vi "SE FP hindbrain SENSE.vi"(0 "IR Sensors":T1(array[cluster]), 1 "Analog Input Values":dbl[](array[numeric]), 2 "error in":errorcluster, 4 "GPS":cluster{"X pos":i32, "Y pos":i32, "Heading":dbl}) -> (3 "Boat Status":T2, 5 "error out":errorcluster, 6 "IR Sensors 2":T1(array[cluster]))   [LabVIEW 2014]
doc: "This vi calculate the distance from the boat edge to the detected object. If no object is detected the value is 0. It also determines of the boat is out of power...if so it will stop the boat."
panel:
  out "RIO BAT":dbl
  out "MOT BAT":dbl
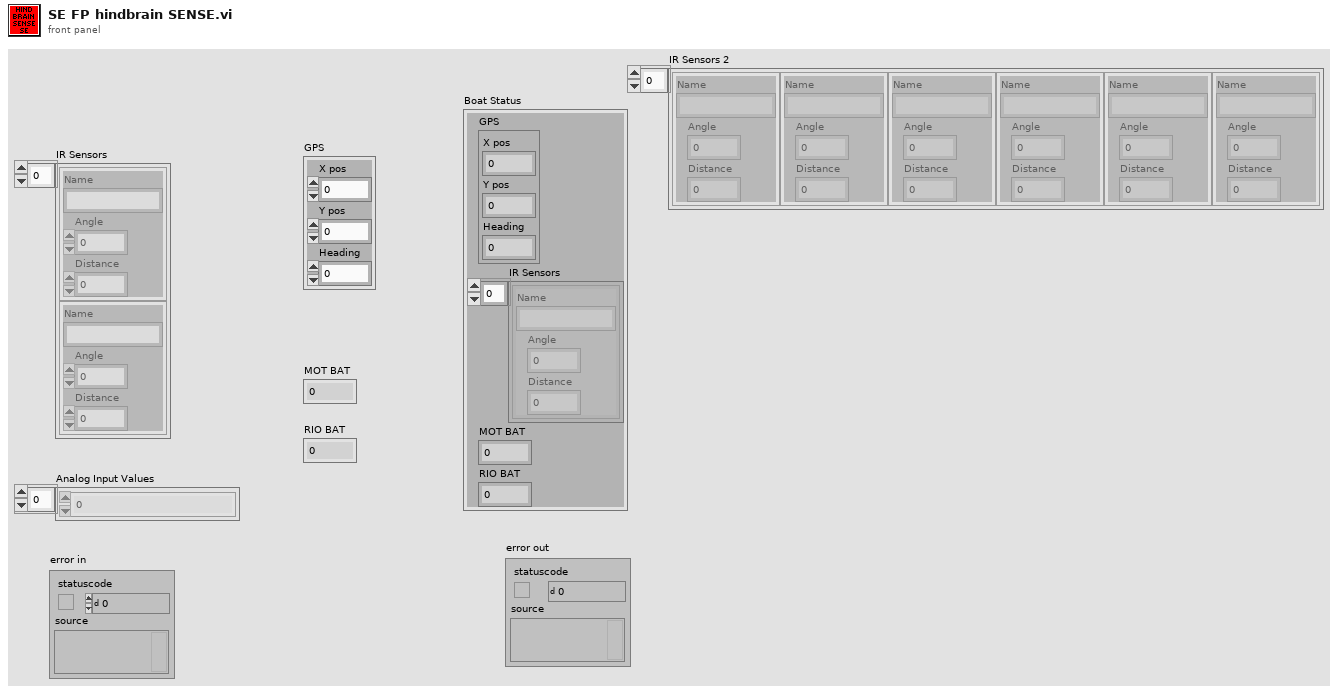
[diagram p1: front panel]
types:
  T1 = cluster{"Name":string, "Angle":dbl, "Distance":dbl}[]
  T2 = cluster{"GPS":cluster{"X pos":i32, "Y pos":i32, "Heading":dbl}, "IR Sensors":cluster{"Name":string, "Angle":dbl, "Distance":dbl}[], "MOT BAT":dbl, "RIO BAT":dbl}
  T3 = cluster{"Name":string, "Angle":dbl, "Distance":dbl}
  T4 = cluster{"GPS":cluster{"X pos":i32, "Y pos":i32, "Heading":dbl}, cluster{"Name":string, "Angle":dbl, "Distance":dbl}[], "MOT BAT":dbl, "RIO BAT":dbl}
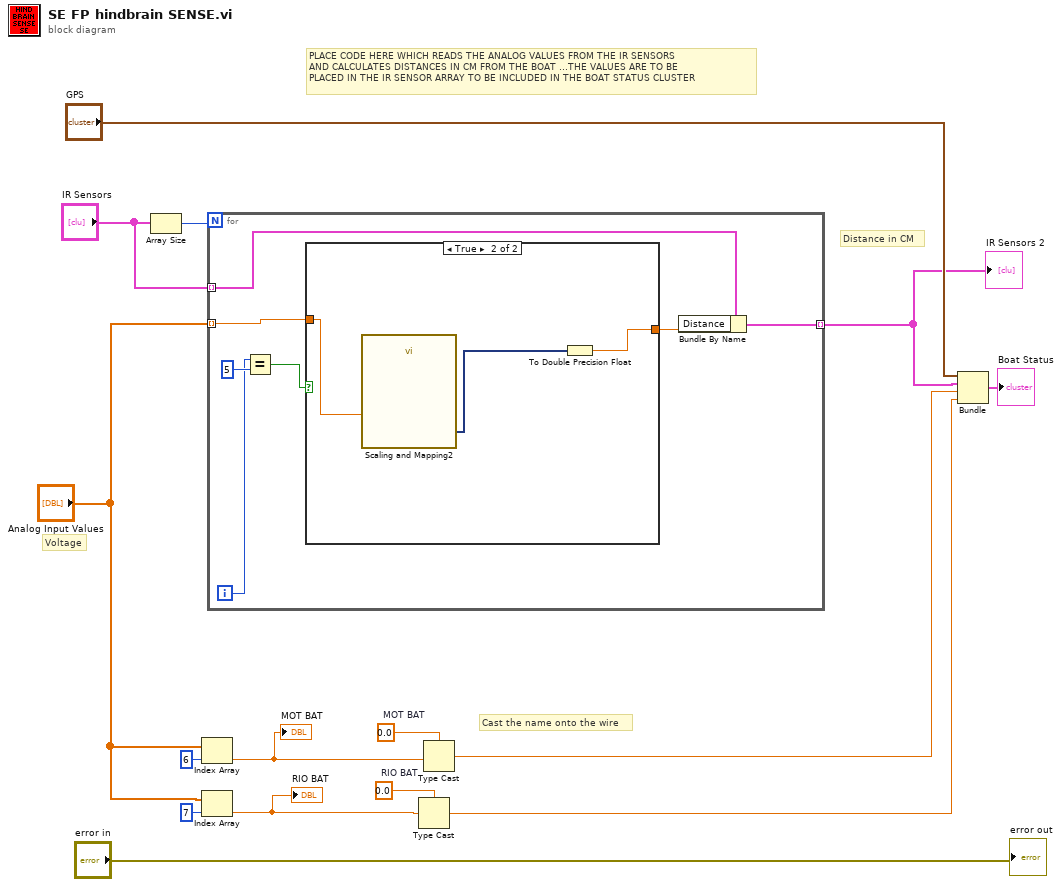
[diagram p0: block diagram]
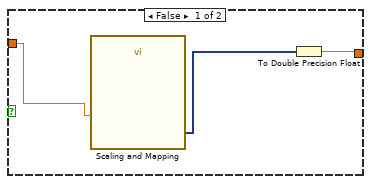
[diagram p2: hidden frame]
diagram:
  w8 = 0.0  # RIO BAT
  w12 = 0.0  # MOT BAT
  # "Voltage"
  # "Distance in CM"
  # "PLACE CODE HERE WHICH READS THE ANALOG VALUES FROM THE IR SENSORS \nAND CALCULATES DISTANCES IN CM FROM THE BOAT ...THE VALUES ARE TO BE \nPLACED IN THE IR SENSOR ARRAY TO BE INCLUDED IN THE BOAT STATUS CLUSTER"
  # "Cast the name onto the wire"
  n1 = Array Size(array="IR Sensors") -> (size(s)=w3:i32)
  n2 = Index Array(array="Analog Input Values", index=6) -> (element=w11:dbl)
  "MOT BAT" <- w11
  n3 = Index Array(array="Analog Input Values", index=7) -> (element=w7:dbl)
  "RIO BAT" <- w7
  n4 = for {
    N: w3 -> [_]
    tunnel: "IR Sensors" -> [w20] mode=indexing
    tunnel: "Analog Input Values" -> [w19] mode=indexing
    tunnel: [w22] -> w2 mode=indexing
    i -> [w16]
    n5 = Equal?(x=w16, y=5) -> (x = y?=w18:bool)
    n6 = case shown="True" w18 {
      tunnel: [w25 w28] -> w21
      tunnel: w19 -> [w24 w26]
      frame False {
        n7 = call "Scaling and Mapping"("Signals"=w24) -> ("Scaled Signals"=w23:dynamicdata)  [unwired: 9 in, 1 out]
        n8 = To Double Precision Float(number=w23) -> (double precision float=w25:dbl)
      }
      frame True {
        n9 = call "Scaling and Mapping2"("Signals"=w26) -> ("Scaled Signals"=w27:dynamicdata)  [unwired: 9 in, 1 out]
        n10 = To Double Precision Float(number=w27) -> (double precision float=w28:dbl)
      }
    }
    n11 = Bundle By Name(cluster=w20, "Distance"=w21) -> (w22:T3)
  }
  "IR Sensors 2" <- w2
  n12 = Type Cast(type=w8, x=w7) -> (*(type *) &x=w6:dbl)
  n13 = Type Cast(type=w12, x=w11) -> (*(type *) &x=w10:dbl)
  n14 = Bundle("GPS"="GPS", w2, "MOT BAT"=w10, "RIO BAT"=w6) -> (→"Boat Status":T4)  [unwired: 1 in]
  "error out" <- "error in"
